vi "_Parse SEM Margin Area Results.vi"(8 "error in (no error)":errorcluster, 10 "Input String":string, 11 "VISA resource name":refnum<visa-resource-name>) -> (0 "error out":errorcluster, 1 "Results":cluster{"Margin X":dbl, "Margin Y":dbl}[](array[cluster]), 2 "Reliability":i32, 3 "VISA resource name out":refnum<visa-resource-name>)   [LabVIEW 2020, in "Rohde&Schwarz CMWXP NR FR1 Measurement.lvlib"]
uses:
  <instrlib>/Rohde&Schwarz CMWXP NR FR1 Measurement/Rohde&Schwarz CMWXP NR FR1 Measurement.lvlib
  <instrlib>/Rohde&Schwarz CMWXP NR FR1 Measurement/Private/rsidr_core.llb/rsidr_core.lvlib
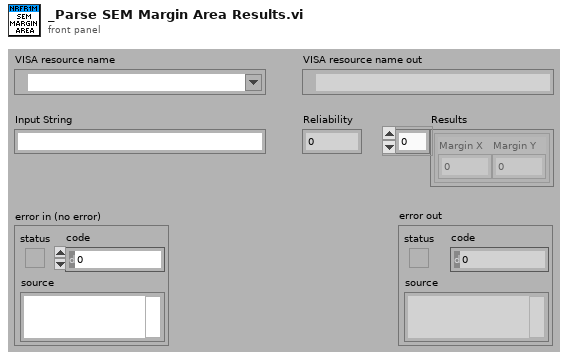
[diagram p1: front panel]
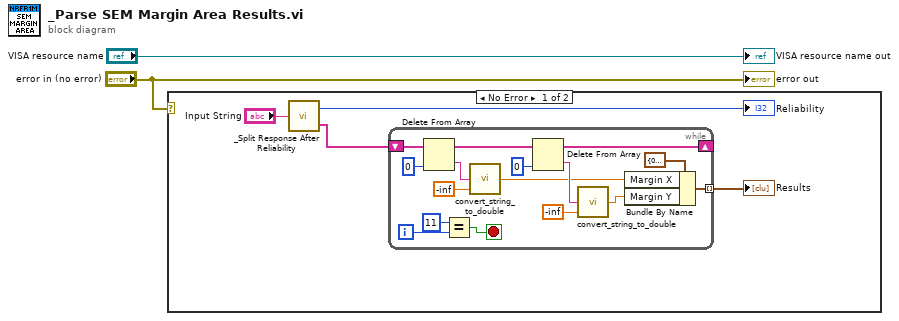
[diagram p0: block diagram]
diagram:
  n1 = case shown="No Error" "error in (no error)" {
    frame No Error {
      n2 = call <instrlib>:"_Split Response After Reliability.vi"("Input String"="Input String") -> ("Response out"=w3:string[], "Reliability out"=→"Reliability":i32)
      n3 = while {
        shift-right: [w13] -> _
        shift-left: w3 -> [w20]
        tunnel: [w7] -> w4 mode=indexing
        i -> [w10]
        stop <- w9 stop-if-true
        n4 = Delete From Array(array=w20, index=0) -> (deleted portion=w22:string, array with subset deleted=w16:string[])  [unwired: 1 in]
        n5 = Equal?(x=11, y=w10) -> (x = y?=w9:bool)
        n6 = call <instrlib>:"convert_string_to_double.vi"("default (0)"=-inf, "String in"=w22) -> ("double value out"=w15:dbl)  [unwired: 3 in]
        n7 = Delete From Array(array=w16, index=0) -> (deleted portion=w17:string, array with subset deleted=w13:string[])  [unwired: 1 in]
        n8 = call <instrlib>:"convert_string_to_double.vi"("default (0)"=-inf, "String in"=w17) -> ("double value out"=w14:dbl)  [unwired: 3 in]
        n9 = Bundle By Name(cluster=cluster{"Margin X":dbl, "Margin Y":dbl} {"Margin X"=0.0, "Margin Y"=0.0} ("X and Y Value Pair"), "Margin X"=w15, "Margin Y"=w14) -> (w7:cluster{"Margin X":dbl, "Margin Y":dbl})
      }
      "Results" <- w4
    }
    frame Error {
    }
  }
  "error out" <- "error in (no error)"
  "VISA resource name out" <- "VISA resource name"
